vi "Get Multiple Tags.vi"(8 "error in (no error)":errorcluster, 10 "Cluster":variant, 11 "uData in":refnum<class "uData.lvclass">) -> (0 "error out":errorcluster, 2 "data":variant, 3 "uData out":refnum<class "uData.lvclass">, 4 "all found?":bool, 6 "found tags":string[](array[string]))   [LabVIEW 2023, in "uLib.lvlib" / "uData.lvclass"]
doc: "Wire in a cluster with <B>LABELLED</B> elements. The cluster will be broken into individual elements, each element is used to read the corresponding tag. \nNested clusters use a label[dot]sublabel notation.\n\nWiring non-cluster datatypes or clusters with unlabelled element will throw out a runtime error.\n\nDo NOT use for handling data at high rates. This VI does not support inlining and has a high overhead due to data type conversion. Use only when convenience is required for generic messaging. However, the basic accessor methods are more efficient for recurring high rate VI calls"
uses:
  uData.lvclass
  uData.lvclass/uData.ctl
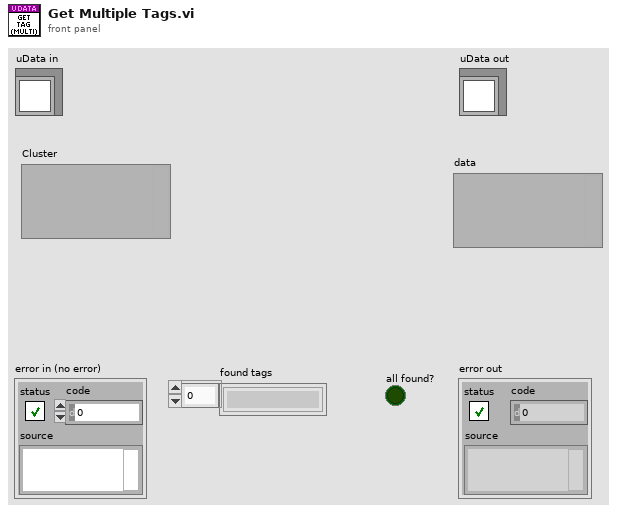
[diagram p1: front panel]
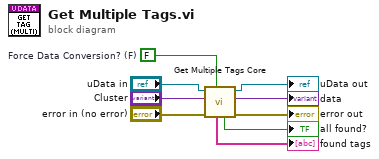
[diagram p0: block diagram]
diagram:
  w1 = FALSE  # Force Data Conversion? (F)
  n1 = call "Get Multiple Tags Core.vi"("Force Data Conversion? (F)"=w1, "error in (no error)"="error in (no error)", "Cluster"="Cluster", "uData in"="uData in") -> ("error out"=→"error out":errorcluster, "data"=→"data":variant, "uData out"=→"uData out":refnum<class "uData.lvclass">, "all found?"=→"all found?":bool, "found tags"=→"found tags":string[])  [unwired: 3 in]
